vi "FieldCentricCalc.vi"(9 "RobotFront":bool, 10 "y_in":dbl, 11 "x_in":dbl) -> (2 "y_out":dbl, 3 "x_out":dbl)   [LabVIEW 2018]
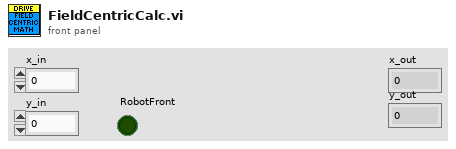
[diagram p1: front panel]
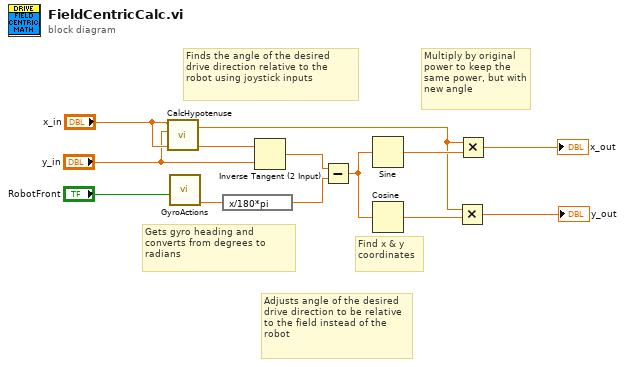
[diagram p0: block diagram]
diagram:
  # "Multiply by original power to keep the same power, but with new angle"
  # "Adjusts angle of the desired drive direction to be relative to the field instead of the robot"
  # "Find x & y coordinates"
  # "Gets gyro heading and converts from degrees to radians"
  # "Finds the angle of the desired drive direction relative to the robot using joystick inputs"
  n1 = call "CalcHypotenuse.vi"("b"="y_in", "a"="x_in") -> ("hypotenuse"=w2:dbl)  [unwired: 3 in]
  n2 = call "GyroActions.vi"("RobotFront"="RobotFront") -> ("Yaw"=w8:dbl)  [unwired: 9 in, 1 out]
  n3 = expression code="x/180*pi"(w8) -> (w6:dbl)
  n4 = Inverse Tangent (2 Input)(1:"y_in", 2:"x_in") -> (0:w7:dbl)
  n5 = Subtract(x=w7, y=w6) -> (x-y=w5:dbl)
  n6 = Sine(x=w5) -> (sin(x)=w3:dbl)
  n7 = Cosine(x=w5) -> (cos(x)=w4:dbl)
  n8 = Multiply(x=w2, y=w4) -> (x*y=→"y_out":dbl)
  n9 = Multiply(x=w2, y=w3) -> (x*y=→"x_out":dbl)
